vi "Write T Controller Settings.vi"(4 "New PID":cluster{"P":dbl, "I":dbl, "D":dbl}, 6 "Heater level":dbl, 7 "Set point":dbl, 8 "error in (no error)":errorcluster, 9 "New Heater mode":T1(ring), 10 "Heater range":dbl, 11 "LakeShore 340 in":refnum<class "LakeShore 340.lvclass">) -> (0 "error out":errorcluster, 3 "LakeShore 340 out":refnum<class "LakeShore 340.lvclass">)   [LabVIEW 2015, in "LakeShore 340.lvclass"]
uses:
  LakeShore 340.lvclass
  Instrument/Instrument.lvclass
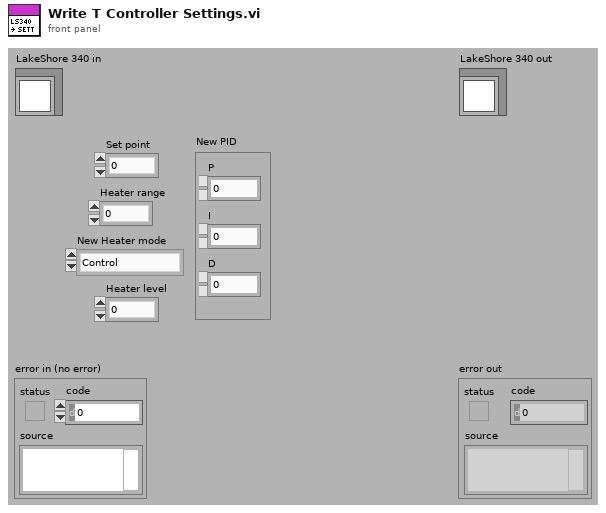
[diagram p1: front panel]
types:
  T1 = enum16{"Control", "Monitor", "Manual Heat", "Controller is in OFF mode", "Autotune is in progress"}
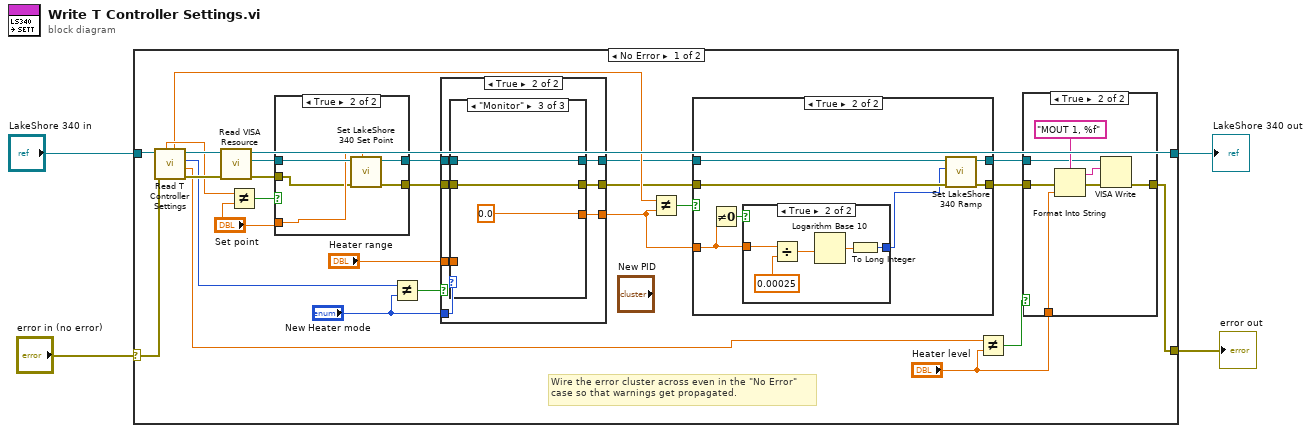
[diagram p0: block diagram]
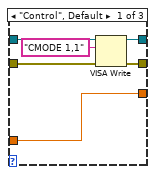
[diagram p4: hidden frame]
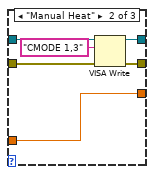
[diagram p5: hidden frame]
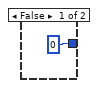
[diagram p7: hidden frame]
diagram:
  n1 = case shown="No Error" "error in (no error)" {
    selector: "error in (no error)" -> [w27 w88]
    tunnel: [w5 w88] -> w3
    tunnel: [w30 w87] -> w1
    tunnel: "LakeShore 340 in" -> [w31 w87]
    frame No Error {
      # "Wire the error cluster across even in the \"No Error\"\ncase so that warnings get propagated."
      n2 = call-dynamic "Read T Controller Settings.vi"("error in (no error)"=w27, "LakeShore 340 in"=w31) -> ("error out"=w28:errorcluster, "Heater level"=w10:dbl, "Heater mode"=w19:T1, "LakeShore 340 out"=w29:refnum<class "LakeShore 340.lvclass">, "Hater range"=w20:dbl, "Set point"=w26:dbl)  [unwired: 4 out]
      n3 = call "Read VISA Resource.vi"("error in (no error)"=w28, "Instrument.lvclass in"=w29) -> ("error out"=w24:errorcluster, "VISA Resource"=w22:refnum<visa-resource-name>, "Instrument.lvclass out"=w30:refnum<class "LakeShore 340.lvclass">)  [unwired: 7 out]
      n4 = Not Equal?(x=w26, y="Set point") -> (x != y?=w25:bool)
      n5 = case shown="True" w25 {
        tunnel: w24 -> [w81 w82]
        tunnel: "Set point" -> [_ w83]
        tunnel: w22 -> [w80 w86]
        tunnel: [w81 w85] -> w14
        tunnel: [w80 w84] -> w13
        frame False {
        }
        frame True {
          n6 = call "Set LakeShore 340 Set Point.vi"("Set point"=w83, "error in (no error)"=w82, "VISA Resource Name"=w86) -> ("error out"=w85:errorcluster, "VISA Resource Name Out"=w84:refnum<visa-resource-name>)  [unwired: 7 in]
        }
      }
      n7 = Not Equal?(x=w19, y="New Heater mode") -> (x != y?=w18:bool)
      n8 = case shown="True" w18 {
        tunnel: "New Heater mode" -> [_ w49]
        tunnel: "Heater range" -> [w42 w48]
        tunnel: [w42 w47] -> w15
        tunnel: w14 -> [w41 w46]
        tunnel: w13 -> [w40 w45]
        tunnel: [w40 w44] -> w11
        tunnel: [w41 w43] -> w12
        frame False {
        }
        frame True {
          n9 = case shown="\"Monitor\"" w49 {
            tunnel: w48 -> [w55 w61 _]
            tunnel: [w55 w61 0.0 ("Heater range")] -> w47
            tunnel: w46 -> [w54 w60 w63]
            tunnel: w45 -> [w53 w59 w62]
            tunnel: [w51 w57 w63] -> w43
            tunnel: [w50 w56 w62] -> w44
            frame "Control", Default {
              n10 = VISA Write(VISA resource name=w53, write buffer="CMODE 1,1", error in (no error)=w54) -> (VISA resource name out=w50:refnum<visa-resource-name>, error out=w51:errorcluster)  [unwired: 1 out]
            }
            frame "Manual Heat" {
              n11 = VISA Write(VISA resource name=w59, write buffer="CMODE 1,3", error in (no error)=w60) -> (VISA resource name out=w56:refnum<visa-resource-name>, error out=w57:errorcluster)  [unwired: 1 out]
            }
            frame "Monitor" {
            }
          }
        }
      }
      n12 = Not Equal?(x=w20, y=w15) -> (x != y?=w21:bool)
      n13 = case shown="True" w21 {
        tunnel: w12 -> [w66 w68]
        tunnel: w15 -> [_ w69]
        tunnel: w11 -> [w65 w73]
        tunnel: [w66 w72] -> w7
        tunnel: [w65 w71] -> w8
        frame False {
        }
        frame True {
          n14 = Not Equal To 0?(x=w69) -> (x != 0?=w70:bool)
          n15 = case shown="True" w70 {
            tunnel: w69 -> [_ w78]
            tunnel: [0 w75] -> w67
            frame False {
            }
            frame True {
              n16 = Divide(x=w78, y=0.00025) -> (x/y=w77:dbl)
              n17 = Logarithm Base 10(1:w77) -> (0:w76:dbl)
              n18 = To Long Integer(number=w76) -> (32bit integer=w75:i32)
            }
          }
          n19 = call "Set LakeShore 340 Ramp.vi"("error in (no error)"=w68, "Approach"=w67, "VISA resource name"=w73) -> ("error out"=w72:errorcluster, "VISA resource name out"=w71:refnum<visa-resource-name>)  [unwired: 7 in]
        }
      }
      n20 = Not Equal?(x=w10, y="Heater level") -> (x != y?=w9:bool)
      n21 = case shown="True" w9 {
        tunnel: w8 -> [_ w34]
        tunnel: w7 -> [w32 w35]
        tunnel: "Heater level" -> [_ w36]
        tunnel: [w32 w33] -> w5
        frame False {
        }
        frame True {
          n22 = Format Into String(format string="MOUT 1, %f" ("write buffer"), error in=w35, w36) -> (resulting string=w37:string, error out=w38:errorcluster)  [unwired: 1 in]
          n23 = VISA Write(VISA resource name=w34, write buffer=w37, error in (no error)=w38) -> (error out=w33:errorcluster)  [unwired: 2 out]
        }
      }
    }
    frame Error {
    }
  }
  "error out" <- w3
  "LakeShore 340 out" <- w1
